vi "DisplayGraph.vi"(3 "error in (no error)":errorcluster, 4 "Amplitude":dbl=1.0, 5 "Frequency":dbl=10.1) -> (0 "array":dynamicdata[](array[waveform]), 1 "error out":errorcluster)   [LabVIEW 2011]
uses:
  Instance           1 20Saved   DisplayGraph .vi
panel:
  in  "stop":bool
  out "Waveform Chart":dynamicdata(graph)
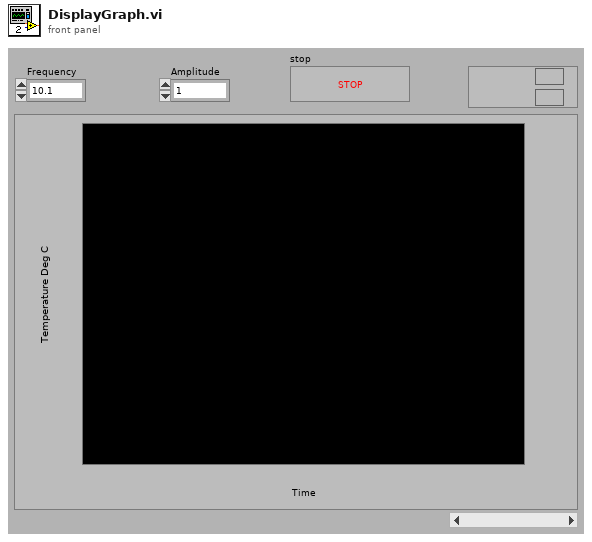
[diagram p1: front panel]
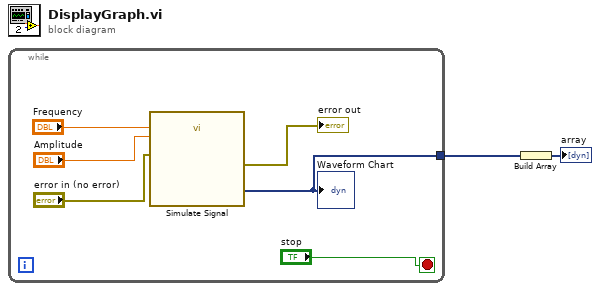
[diagram p0: block diagram]
diagram:
  n1 = while {
    tunnel: [w3] -> w2
    stop <- "stop" stop-if-true
    n2 = call "Simulate Signal"("Frequency"="Frequency", "Amplitude"="Amplitude", "error in (no error)"="error in (no error)") -> ("Sine"=w3:dynamicdata, "error out"=→"error out":errorcluster)  [unwired: 3 in, 8 out]
    "Waveform Chart" <- w3
  }
  n3 = Build Array(w2) -> (→"array":dynamicdata[])
